vi "Activity_14.vi"() -> ()   [LabVIEW 2015]
panel:
  in  "stop":bool
  out "Boolean 5":bool
  out "Boolean 4":bool
  out "Boolean 3":bool
  out "Boolean 2":bool
  out "Boolean":bool
  out "Terminal1":string
  out "Terminal2":string
  out "Terminal3":string
  out "Terminal4":string
  out "Terminal5":string
  out "Destino2":string
  out "Destino5":string
  out "Destino4":string
  out "Destino3":string
  out "Destino1":string
  out "Aerolinea5":u16(ring)
  out "Aerolinea4":u16(ring)
  out "Aerolinea3":u16(ring)
  out "Aerolinea2":u16(ring)
  out "Aerolinea":u16(ring)
  out "Titulo":string
  out "Titulo2":string
  # "Simulador de Tablero de Anuncios de Vuelo"
  # "Serrano Bermúdez Luis Esteban\nFecha de Entrega 02/03/2019"
  # "Descripción:"
  # "Simula la llegada y salida de vuelos en un Aeropuerto, muestra\nel destino, la aerolinea, el estatus del vuelo y la terminal del vuelo\nHace un restraso de 5 seg. entre cada cambio de estado. Este modelo\nusa una maquina de estados"
  # "Destino"
  # "Terminal"
  # "Aerolinea"
  # "Estatus"
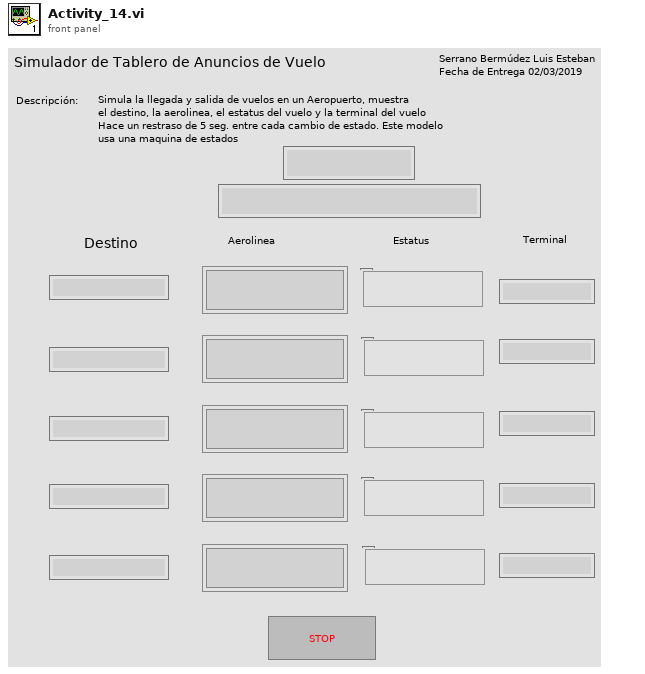
[diagram p1: front panel]
types:
  T1 = enum16{"LlegNac", "LlegInter", "SalNac", "SalInter"}
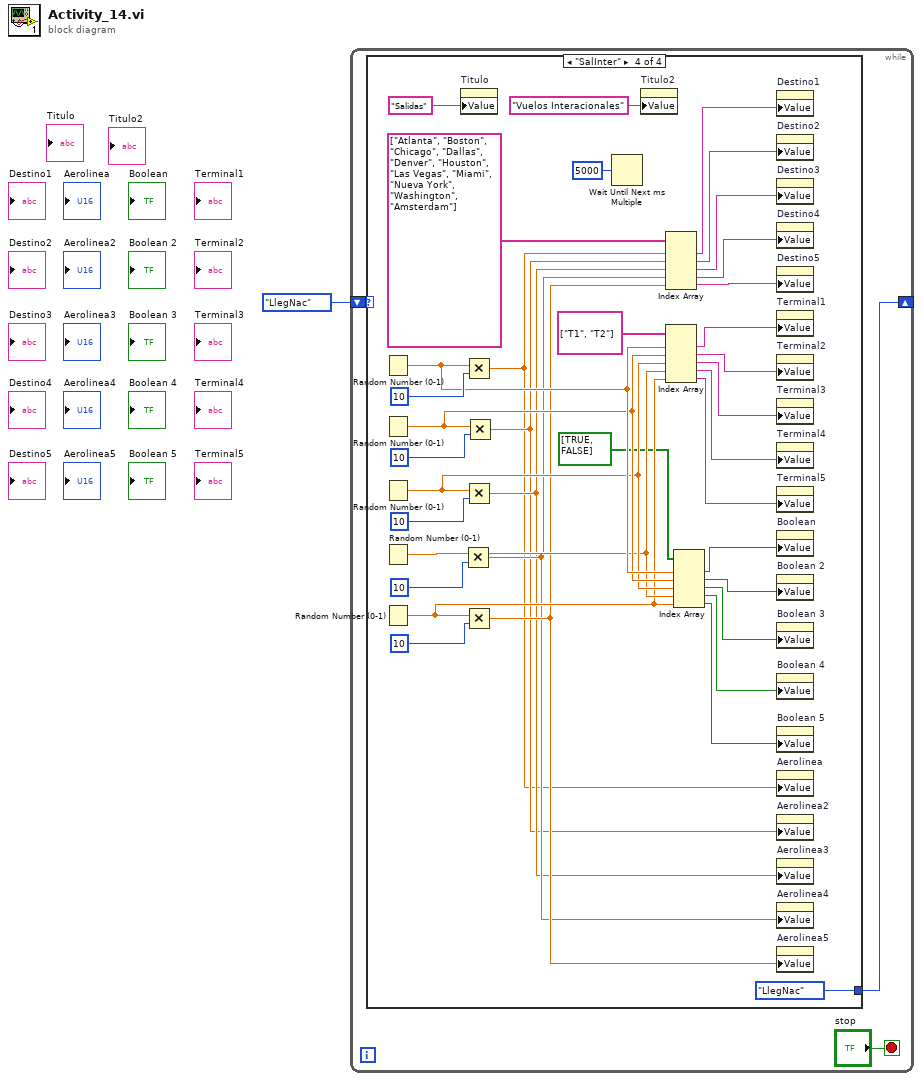
[diagram p0: block diagram]
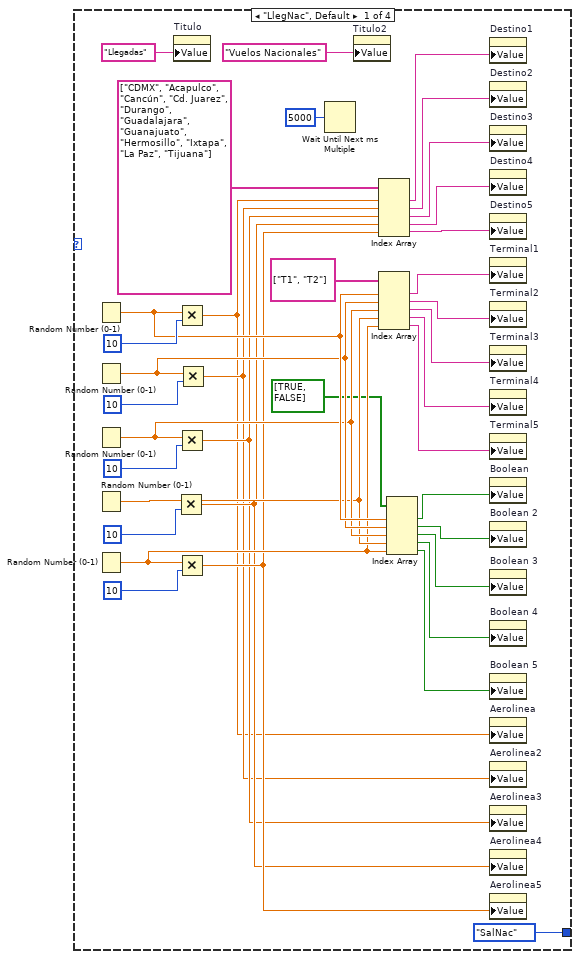
[diagram p2: hidden frame]
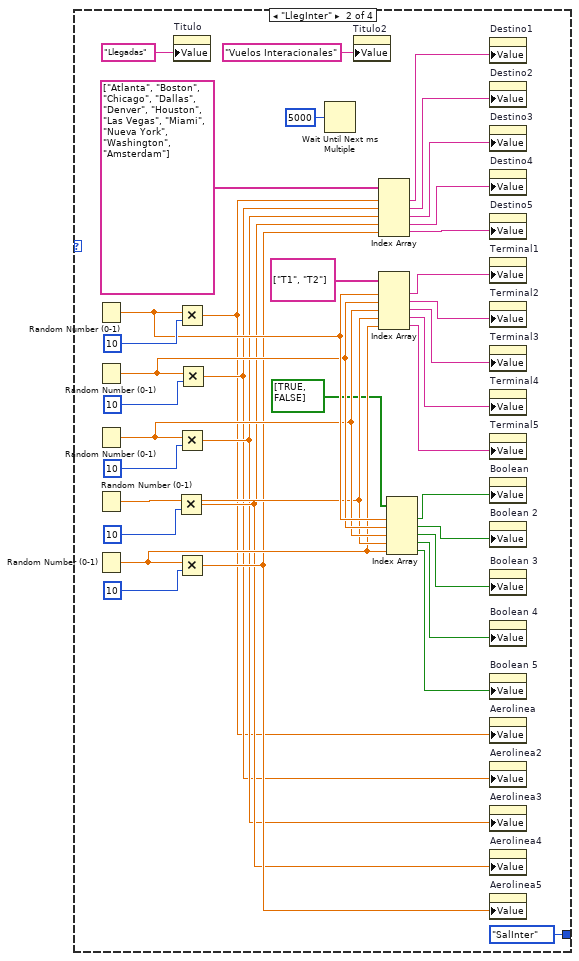
[diagram p3: hidden frame]
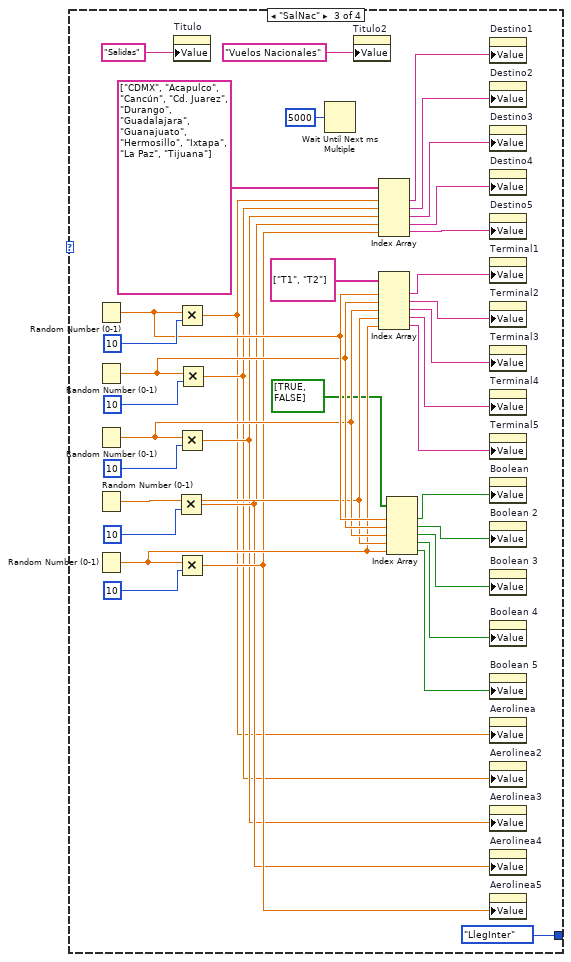
[diagram p4: hidden frame]
diagram:
  n1 = while {
    shift-right: [w3] -> _
    shift-left: T1."LlegNac" -> [w4]
    stop <- "stop" stop-if-true
    n2 = case shown="\"SalInter\"" w4 {
      tunnel: [T1."SalNac" T1."SalInter" T1."LlegInter" T1."LlegNac"] -> w3
      frame "LlegNac", Default {
        n3 = Random Number (0-1)() -> (number: 0 to 1=w33:dbl)
        n4 = Random Number (0-1)() -> (number: 0 to 1=w32:dbl)
        n5 = Random Number (0-1)() -> (number: 0 to 1=w31:dbl)
        n6 = Random Number (0-1)() -> (number: 0 to 1=w30:dbl)
        n7 = Random Number (0-1)() -> (number: 0 to 1=w29:dbl)
        n8 = property on="Titulo" class="Str"("Value"="Llegadas") -> ()  [unwired: 2 in, 2 out]
        n9 = Multiply(x=w30, y=10) -> (x*y=w9:dbl)
        n10 = Multiply(x=w33, y=10) -> (x*y=w6:dbl)
        n11 = Multiply(x=w31, y=10) -> (x*y=w8:dbl)
        n12 = Multiply(x=w29, y=10) -> (x*y=w10:dbl)
        n13 = Multiply(x=w32, y=10) -> (x*y=w7:dbl)
        n14 = Wait Until Next ms Multiple(millisecond multiple=u32 5000) -> ()  [unwired: 1 out]
        n15 = property on="Titulo2" class="Str"("Value"="Vuelos Nacionales") -> ()  [unwired: 2 in, 2 out]
        n16 = Index Array(array=string[] ["CDMX", "Acapulco", "Cancún", "Cd. Juarez", "Durango", "Guadalajara", "Guanajuato", "Hermosillo", "Ixtapa", "La Paz", "Tijuana"], index #1=w6, index #2=w7, index #3=w8, index #4=w9, index #5=w10) -> (element #1=w25:string, element #2=w24:string, element #3=w23:string, element #4=w22:string, element #5=w21:string)
        n17 = Index Array(array=string[] ["T1", "T2"], index #1=w33, index #2=w32, index #3=w31, index #4=w30, index #5=w29) -> (element #1=w20:string, element #2=w19:string, element #3=w18:string, element #4=w17:string, element #5=w16:string)
        n18 = Index Array(array=bool[] [TRUE, FALSE], index #1=w33, index #2=w32, index #3=w31, index #4=w30, index #5=w29) -> (element #1=w15:bool, element #2=w14:bool, element #3=w13:bool, element #4=w12:bool, element #5=w11:bool)
        n19 = property on="Destino1" class="Str"("Value"=w25) -> ()  [unwired: 2 in, 2 out]
        n20 = property on="Destino2" class="Str"("Value"=w24) -> ()  [unwired: 2 in, 2 out]
        n21 = property on="Destino3" class="Str"("Value"=w23) -> ()  [unwired: 2 in, 2 out]
        n22 = property on="Destino4" class="Str"("Value"=w22) -> ()  [unwired: 2 in, 2 out]
        n23 = property on="Destino5" class="Str"("Value"=w21) -> ()  [unwired: 2 in, 2 out]
        n24 = property on="Terminal1" class="Str"("Value"=w20) -> ()  [unwired: 2 in, 2 out]
        n25 = property on="Terminal2" class="Str"("Value"=w19) -> ()  [unwired: 2 in, 2 out]
        n26 = property on="Terminal3" class="Str"("Value"=w18) -> ()  [unwired: 2 in, 2 out]
        n27 = property on="Terminal4" class="Str"("Value"=w17) -> ()  [unwired: 2 in, 2 out]
        n28 = property on="Terminal5" class="Str"("Value"=w16) -> ()  [unwired: 2 in, 2 out]
        n29 = property on="Boolean" class="Bool (strict)"("Value"=w15) -> ()  [unwired: 2 in, 2 out]
        n30 = property on="Boolean 2" class="Bool (strict)"("Value"=w14) -> ()  [unwired: 2 in, 2 out]
        n31 = property on="Boolean 3" class="Bool (strict)"("Value"=w13) -> ()  [unwired: 2 in, 2 out]
        n32 = property on="Boolean 4" class="Bool (strict)"("Value"=w12) -> ()  [unwired: 2 in, 2 out]
        n33 = property on="Boolean 5" class="Bool (strict)"("Value"=w11) -> ()  [unwired: 2 in, 2 out]
        n34 = property on="Aerolinea" class="Ring (strict)"("Value"=w6) -> ()  [unwired: 2 in, 2 out]
        n35 = property on="Aerolinea2" class="Ring (strict)"("Value"=w7) -> ()  [unwired: 2 in, 2 out]
        n36 = property on="Aerolinea3" class="Ring (strict)"("Value"=w8) -> ()  [unwired: 2 in, 2 out]
        n37 = property on="Aerolinea4" class="Ring (strict)"("Value"=w9) -> ()  [unwired: 2 in, 2 out]
        n38 = property on="Aerolinea5" class="Ring (strict)"("Value"=w10) -> ()  [unwired: 2 in, 2 out]
      }
      frame "LlegInter" {
        n39 = Random Number (0-1)() -> (number: 0 to 1=w70:dbl)
        n40 = Random Number (0-1)() -> (number: 0 to 1=w69:dbl)
        n41 = Random Number (0-1)() -> (number: 0 to 1=w68:dbl)
        n42 = Random Number (0-1)() -> (number: 0 to 1=w67:dbl)
        n43 = Random Number (0-1)() -> (number: 0 to 1=w66:dbl)
        n44 = property on="Titulo" class="Str"("Value"="Llegadas") -> ()  [unwired: 2 in, 2 out]
        n45 = Multiply(x=w67, y=10) -> (x*y=w46:dbl)
        n46 = Multiply(x=w70, y=10) -> (x*y=w43:dbl)
        n47 = Multiply(x=w68, y=10) -> (x*y=w45:dbl)
        n48 = Multiply(x=w66, y=10) -> (x*y=w47:dbl)
        n49 = Multiply(x=w69, y=10) -> (x*y=w44:dbl)
        n50 = Wait Until Next ms Multiple(millisecond multiple=u32 5000) -> ()  [unwired: 1 out]
        n51 = property on="Titulo2" class="Str"("Value"="Vuelos Interacionales") -> ()  [unwired: 2 in, 2 out]
        n52 = Index Array(array=string[] ["Atlanta", "Boston", "Chicago", "Dallas", "Denver", "Houston", "Las Vegas", "Miami", "Nueva York", "Washington", "Amsterdam"], index #1=w43, index #2=w44, index #3=w45, index #4=w46, index #5=w47) -> (element #1=w62:string, element #2=w61:string, element #3=w60:string, element #4=w59:string, element #5=w58:string)
        n53 = Index Array(array=string[] ["T1", "T2"], index #1=w70, index #2=w69, index #3=w68, index #4=w67, index #5=w66) -> (element #1=w57:string, element #2=w56:string, element #3=w55:string, element #4=w54:string, element #5=w53:string)
        n54 = Index Array(array=bool[] [TRUE, FALSE], index #1=w70, index #2=w69, index #3=w68, index #4=w67, index #5=w66) -> (element #1=w52:bool, element #2=w51:bool, element #3=w50:bool, element #4=w49:bool, element #5=w48:bool)
        n55 = property on="Destino1" class="Str"("Value"=w62) -> ()  [unwired: 2 in, 2 out]
        n56 = property on="Destino2" class="Str"("Value"=w61) -> ()  [unwired: 2 in, 2 out]
        n57 = property on="Destino3" class="Str"("Value"=w60) -> ()  [unwired: 2 in, 2 out]
        n58 = property on="Destino4" class="Str"("Value"=w59) -> ()  [unwired: 2 in, 2 out]
        n59 = property on="Destino5" class="Str"("Value"=w58) -> ()  [unwired: 2 in, 2 out]
        n60 = property on="Terminal1" class="Str"("Value"=w57) -> ()  [unwired: 2 in, 2 out]
        n61 = property on="Terminal2" class="Str"("Value"=w56) -> ()  [unwired: 2 in, 2 out]
        n62 = property on="Terminal3" class="Str"("Value"=w55) -> ()  [unwired: 2 in, 2 out]
        n63 = property on="Terminal4" class="Str"("Value"=w54) -> ()  [unwired: 2 in, 2 out]
        n64 = property on="Terminal5" class="Str"("Value"=w53) -> ()  [unwired: 2 in, 2 out]
        n65 = property on="Boolean" class="Bool (strict)"("Value"=w52) -> ()  [unwired: 2 in, 2 out]
        n66 = property on="Boolean 2" class="Bool (strict)"("Value"=w51) -> ()  [unwired: 2 in, 2 out]
        n67 = property on="Boolean 3" class="Bool (strict)"("Value"=w50) -> ()  [unwired: 2 in, 2 out]
        n68 = property on="Boolean 4" class="Bool (strict)"("Value"=w49) -> ()  [unwired: 2 in, 2 out]
        n69 = property on="Boolean 5" class="Bool (strict)"("Value"=w48) -> ()  [unwired: 2 in, 2 out]
        n70 = property on="Aerolinea" class="Ring (strict)"("Value"=w43) -> ()  [unwired: 2 in, 2 out]
        n71 = property on="Aerolinea2" class="Ring (strict)"("Value"=w44) -> ()  [unwired: 2 in, 2 out]
        n72 = property on="Aerolinea3" class="Ring (strict)"("Value"=w45) -> ()  [unwired: 2 in, 2 out]
        n73 = property on="Aerolinea4" class="Ring (strict)"("Value"=w46) -> ()  [unwired: 2 in, 2 out]
        n74 = property on="Aerolinea5" class="Ring (strict)"("Value"=w47) -> ()  [unwired: 2 in, 2 out]
      }
      frame "SalNac" {
        n75 = Random Number (0-1)() -> (number: 0 to 1=w106:dbl)
        n76 = Random Number (0-1)() -> (number: 0 to 1=w105:dbl)
        n77 = Random Number (0-1)() -> (number: 0 to 1=w104:dbl)
        n78 = Random Number (0-1)() -> (number: 0 to 1=w103:dbl)
        n79 = Random Number (0-1)() -> (number: 0 to 1=w102:dbl)
        n80 = property on="Titulo" class="Str"("Value"="Salidas") -> ()  [unwired: 2 in, 2 out]
        n81 = Multiply(x=w103, y=10) -> (x*y=w82:dbl)
        n82 = Multiply(x=w106, y=10) -> (x*y=w79:dbl)
        n83 = Multiply(x=w104, y=10) -> (x*y=w81:dbl)
        n84 = Multiply(x=w102, y=10) -> (x*y=w83:dbl)
        n85 = Multiply(x=w105, y=10) -> (x*y=w80:dbl)
        n86 = Wait Until Next ms Multiple(millisecond multiple=u32 5000) -> ()  [unwired: 1 out]
        n87 = property on="Titulo2" class="Str"("Value"="Vuelos Nacionales") -> ()  [unwired: 2 in, 2 out]
        n88 = Index Array(array=string[] ["CDMX", "Acapulco", "Cancún", "Cd. Juarez", "Durango", "Guadalajara", "Guanajuato", "Hermosillo", "Ixtapa", "La Paz", "Tijuana"], index #1=w79, index #2=w80, index #3=w81, index #4=w82, index #5=w83) -> (element #1=w98:string, element #2=w97:string, element #3=w96:string, element #4=w95:string, element #5=w94:string)
        n89 = Index Array(array=string[] ["T1", "T2"], index #1=w106, index #2=w105, index #3=w104, index #4=w103, index #5=w102) -> (element #1=w93:string, element #2=w92:string, element #3=w91:string, element #4=w90:string, element #5=w89:string)
        n90 = Index Array(array=bool[] [TRUE, FALSE], index #1=w106, index #2=w105, index #3=w104, index #4=w103, index #5=w102) -> (element #1=w88:bool, element #2=w87:bool, element #3=w86:bool, element #4=w85:bool, element #5=w84:bool)
        n91 = property on="Destino1" class="Str"("Value"=w98) -> ()  [unwired: 2 in, 2 out]
        n92 = property on="Destino2" class="Str"("Value"=w97) -> ()  [unwired: 2 in, 2 out]
        n93 = property on="Destino3" class="Str"("Value"=w96) -> ()  [unwired: 2 in, 2 out]
        n94 = property on="Destino4" class="Str"("Value"=w95) -> ()  [unwired: 2 in, 2 out]
        n95 = property on="Destino5" class="Str"("Value"=w94) -> ()  [unwired: 2 in, 2 out]
        n96 = property on="Terminal1" class="Str"("Value"=w93) -> ()  [unwired: 2 in, 2 out]
        n97 = property on="Terminal2" class="Str"("Value"=w92) -> ()  [unwired: 2 in, 2 out]
        n98 = property on="Terminal3" class="Str"("Value"=w91) -> ()  [unwired: 2 in, 2 out]
        n99 = property on="Terminal4" class="Str"("Value"=w90) -> ()  [unwired: 2 in, 2 out]
        n100 = property on="Terminal5" class="Str"("Value"=w89) -> ()  [unwired: 2 in, 2 out]
        n101 = property on="Boolean" class="Bool (strict)"("Value"=w88) -> ()  [unwired: 2 in, 2 out]
        n102 = property on="Boolean 2" class="Bool (strict)"("Value"=w87) -> ()  [unwired: 2 in, 2 out]
        n103 = property on="Boolean 3" class="Bool (strict)"("Value"=w86) -> ()  [unwired: 2 in, 2 out]
        n104 = property on="Boolean 4" class="Bool (strict)"("Value"=w85) -> ()  [unwired: 2 in, 2 out]
        n105 = property on="Boolean 5" class="Bool (strict)"("Value"=w84) -> ()  [unwired: 2 in, 2 out]
        n106 = property on="Aerolinea" class="Ring (strict)"("Value"=w79) -> ()  [unwired: 2 in, 2 out]
        n107 = property on="Aerolinea2" class="Ring (strict)"("Value"=w80) -> ()  [unwired: 2 in, 2 out]
        n108 = property on="Aerolinea3" class="Ring (strict)"("Value"=w81) -> ()  [unwired: 2 in, 2 out]
        n109 = property on="Aerolinea4" class="Ring (strict)"("Value"=w82) -> ()  [unwired: 2 in, 2 out]
        n110 = property on="Aerolinea5" class="Ring (strict)"("Value"=w83) -> ()  [unwired: 2 in, 2 out]
      }
      frame "SalInter" {
        n111 = Random Number (0-1)() -> (number: 0 to 1=w144:dbl)
        n112 = Random Number (0-1)() -> (number: 0 to 1=w143:dbl)
        n113 = Random Number (0-1)() -> (number: 0 to 1=w142:dbl)
        n114 = Random Number (0-1)() -> (number: 0 to 1=w141:dbl)
        n115 = Random Number (0-1)() -> (number: 0 to 1=w140:dbl)
        n116 = property on="Titulo" class="Str"("Value"="Salidas") -> ()  [unwired: 2 in, 2 out]
        n117 = Multiply(x=w141, y=10) -> (x*y=w120:dbl)
        n118 = Multiply(x=w144, y=10) -> (x*y=w117:dbl)
        n119 = Multiply(x=w142, y=10) -> (x*y=w119:dbl)
        n120 = Multiply(x=w140, y=10) -> (x*y=w121:dbl)
        n121 = Multiply(x=w143, y=10) -> (x*y=w118:dbl)
        n122 = Wait Until Next ms Multiple(millisecond multiple=u32 5000) -> ()  [unwired: 1 out]
        n123 = property on="Titulo2" class="Str"("Value"="Vuelos Interacionales") -> ()  [unwired: 2 in, 2 out]
        n124 = Index Array(array=string[] ["Atlanta", "Boston", "Chicago", "Dallas", "Denver", "Houston", "Las Vegas", "Miami", "Nueva York", "Washington", "Amsterdam"], index #1=w117, index #2=w118, index #3=w119, index #4=w120, index #5=w121) -> (element #1=w136:string, element #2=w135:string, element #3=w134:string, element #4=w133:string, element #5=w132:string)
        n125 = Index Array(array=string[] ["T1", "T2"], index #1=w144, index #2=w143, index #3=w142, index #4=w141, index #5=w140) -> (element #1=w131:string, element #2=w130:string, element #3=w129:string, element #4=w128:string, element #5=w127:string)
        n126 = Index Array(array=bool[] [TRUE, FALSE], index #1=w144, index #2=w143, index #3=w142, index #4=w141, index #5=w140) -> (element #1=w126:bool, element #2=w125:bool, element #3=w124:bool, element #4=w123:bool, element #5=w122:bool)
        n127 = property on="Destino1" class="Str"("Value"=w136) -> ()  [unwired: 2 in, 2 out]
        n128 = property on="Destino2" class="Str"("Value"=w135) -> ()  [unwired: 2 in, 2 out]
        n129 = property on="Destino3" class="Str"("Value"=w134) -> ()  [unwired: 2 in, 2 out]
        n130 = property on="Destino4" class="Str"("Value"=w133) -> ()  [unwired: 2 in, 2 out]
        n131 = property on="Destino5" class="Str"("Value"=w132) -> ()  [unwired: 2 in, 2 out]
        n132 = property on="Terminal1" class="Str"("Value"=w131) -> ()  [unwired: 2 in, 2 out]
        n133 = property on="Terminal2" class="Str"("Value"=w130) -> ()  [unwired: 2 in, 2 out]
        n134 = property on="Terminal3" class="Str"("Value"=w129) -> ()  [unwired: 2 in, 2 out]
        n135 = property on="Terminal4" class="Str"("Value"=w128) -> ()  [unwired: 2 in, 2 out]
        n136 = property on="Terminal5" class="Str"("Value"=w127) -> ()  [unwired: 2 in, 2 out]
        n137 = property on="Boolean" class="Bool (strict)"("Value"=w126) -> ()  [unwired: 2 in, 2 out]
        n138 = property on="Boolean 2" class="Bool (strict)"("Value"=w125) -> ()  [unwired: 2 in, 2 out]
        n139 = property on="Boolean 3" class="Bool (strict)"("Value"=w124) -> ()  [unwired: 2 in, 2 out]
        n140 = property on="Boolean 4" class="Bool (strict)"("Value"=w123) -> ()  [unwired: 2 in, 2 out]
        n141 = property on="Boolean 5" class="Bool (strict)"("Value"=w122) -> ()  [unwired: 2 in, 2 out]
        n142 = property on="Aerolinea" class="Ring (strict)"("Value"=w117) -> ()  [unwired: 2 in, 2 out]
        n143 = property on="Aerolinea2" class="Ring (strict)"("Value"=w118) -> ()  [unwired: 2 in, 2 out]
        n144 = property on="Aerolinea3" class="Ring (strict)"("Value"=w119) -> ()  [unwired: 2 in, 2 out]
        n145 = property on="Aerolinea4" class="Ring (strict)"("Value"=w120) -> ()  [unwired: 2 in, 2 out]
        n146 = property on="Aerolinea5" class="Ring (strict)"("Value"=w121) -> ()  [unwired: 2 in, 2 out]
      }
    }
  }
